vi "Sound.vi"() -> ()   [LabVIEW 2023]
doc: "This VI illustrates how to acquire sound samples continuously from a specified device. It requires the use of a microphone attached to the sound card. You can specify the number of samples to acquire, sample rate, number of channels and a bit rate per sample. The VI also plots the raw data as the acquisition is made."
uses:
  <vilib>/sound2/lvsound2.llb/Sampling Mode.ctl
  <vilib>/sound2/lvsound2.llb/Sound Data Format.ctl
  <vilib>/sound2/lvsound2.llb/Sound Input Read (DBL).vi
  <vilib>/express/express analysis/Spectral/Block/exnSpectralBlock spectral measurements peak poly.vi
  <vilib>/express/express analysis/Spectral/Block/exnSpectralBlock spectral measurements peak array WFM.vi
  <vilib>/express/express analysis/Spectral/XNode/ExpressSpectralMeasurementsBlockNode.xnode
panel:
  out "Waveform Chart":dbl[](graph)
  out "FFT - (Peak)":cluster{"f0":dbl, "df":dbl, "magnitude":dbl[]}[](array[cluster])
  in  "Device ID":u32 format="%.0x"
  in  "Number of Samples/ch":i32=5000
  out "Raw Data":waveform(dbl)[](graph)
  in  "Stop":bool
  # "Overview: Demonstrates the use of the Sound Input Functions to acquire sound samples continuously with the use of a microphone attached to the sound card.\nRequirements: Microphone\nInstructions:\n1. Specify the Device ID and Number of Samples/ch.\n2. Run the VI.\n3. The VI will continuously acquire samples and plot the raw data to the graph.\n4. Click Stop to stop the VI."
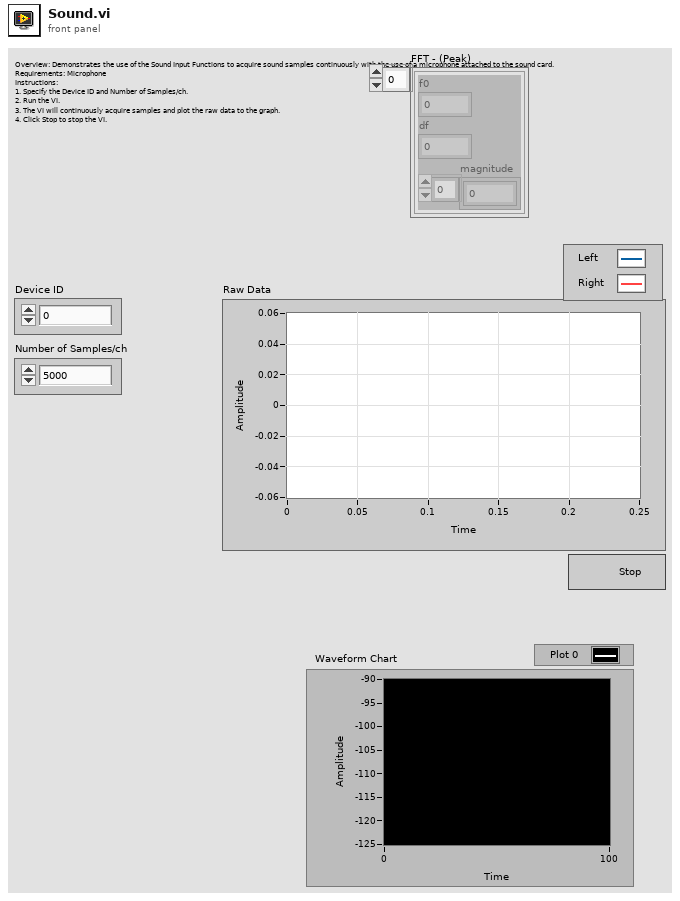
[diagram p1: front panel]
types:
  T1 = typedef "Sound Data Format.ctl" = cluster{"sample rate (S/s)":dbl, "number of channels":i32, "bits per sample":i32}
  T2 = typedef "Sampling Mode.ctl" = i32
  T3 = typedef "Sound Input Task ID.ctl" = u32
  T4 = cluster{"averaging mode":u16, "weighting mode":u16, "number of averages":u32}
  T5 = cluster{"dB On (F)":bool, "unwrap phase (F)":bool, "convert to degree (F)":bool}
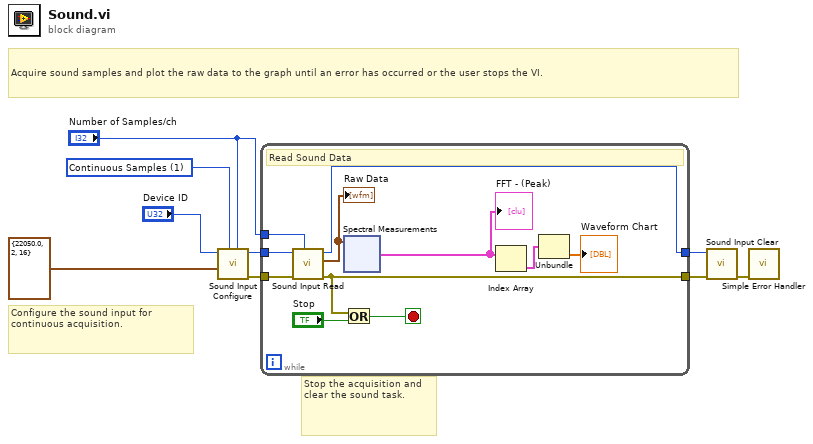
[diagram p0: block diagram]
diagram:
  w4 = T2 1 items=["Finite Samples", "Continuous Samples"] ("sample mode")
  # "Acquire sound samples and plot the raw data to the graph until an error has occurred or the user stops the VI."
  # "Stop the acquisition and clear the sound task."
  # "Configure the sound input for continuous acquisition."
  n1 = call <vilib>:"Sound Input Configure.vi"("number of samples/ch"="Number of Samples/ch", "sample mode"=w4, "sound format"=T1 {"sample rate (S/s)"=22050.0, "number of channels"=2, "bits per sample"=16} ("Sound Format"), "device ID"="Device ID") -> ("error out"=w9:errorcluster, "task ID"=w7:T3)  [unwired: 6 in]
  n2 = while {
    tunnel: w7 -> [w19]
    tunnel: [w18] -> w6
    tunnel: "Number of Samples/ch" -> [w17]
    tunnel: w9 -> [w20]
    tunnel: [w15] -> w5
    stop <- w16 stop-if-true
    # "Read Sound Data"
    n3 = call-poly <vilib>:"Sound Input Read.vi"("number of samples/ch"=w17, "error in (no error)"=w20, "task ID"=w19) -> ("error out"=w15:errorcluster, "data"=w14:waveform(dbl)[], "task ID out"=w18:T3)  [unwired: 6 in]
    "Raw Data" <- w14
    n4 = xnode "Spectral Measurements"("Signals"=w14) -> ("FFT - (Peak)"=w12:cluster{"f0":dbl, "df":dbl, "magnitude":dbl[]}[])  [unwired: 1 in, 2 out]
    "FFT - (Peak)" <- w12
    n5 = Or(x=w15, y="Stop") -> (x .or. y?=w16:bool)
    n6 = Index Array(array=w12) -> (element=w11:cluster{"f0":dbl, "df":dbl, "magnitude":dbl[]})  [unwired: 1 in]
    n7 = Unbundle(w11) -> ("magnitude"=→"Waveform Chart":dbl[])  [unwired: 2 out]
  }
  n8 = call <vilib>:"Sound Input Clear.vi"("error in (no error)"=w5, "task ID"=w6) -> ("error out"=w2:errorcluster)  [unwired: 9 in]
  n9 = call <vilib>:"Simple Error Handler.vi"("error in (no error)"=w2) -> ()  [unwired: 4 in, 5 out]
